vi "queue client testing.vi"() -> ()   [LabVIEW 2015]
uses:
  connection/connection maintainer.lvclass
  message/communicator message.lvclass
  Queue connection/queue pair.ctl
  message/communicator message.lvclass/communicator message.ctl
  communicator/communicator.lvclass/communicator.ctl
  Queue Client/opening handshake data.ctl
  Queue Client/Queue client.lvclass
  Queue connection/Queue connection.lvclass
  communicator/communicator.lvclass
panel:
  out "data 4":variant
  out "ID 4":string
  out "data 3":variant
  out "ID 3":string
  out "conn":refnum<class "connection maintainer.lvclass">
  out "error out 2":errorcluster
  out "listen error":errorcluster
  in  "read queue":bool
  in  "close connn":bool
  in  "listen":bool
  out "error out 4":errorcluster
  out "error out":errorcluster
  in  "send queue":bool
  in  "data 2":string
  in  "ID 2":string
  in  "data":string
  in  "ID":string
  in  "stop":bool
  in  "send handler":bool
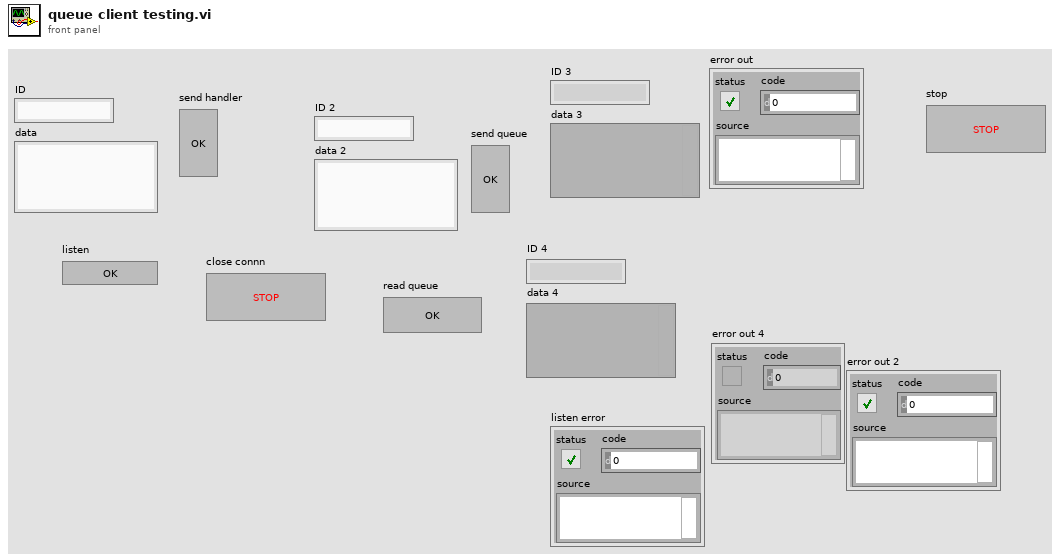
[diagram p1: front panel]
types:
  T1 = typedef "Queue connection.lvclass/queue pair.ctl" = cluster{"to pair":refnum<queue>, "from pair":refnum<queue>}
  T2 = typedef "Queue client.lvclass/opening handshake data.ctl" = cluster{"queue":refnum<queue>, "process ID":string}
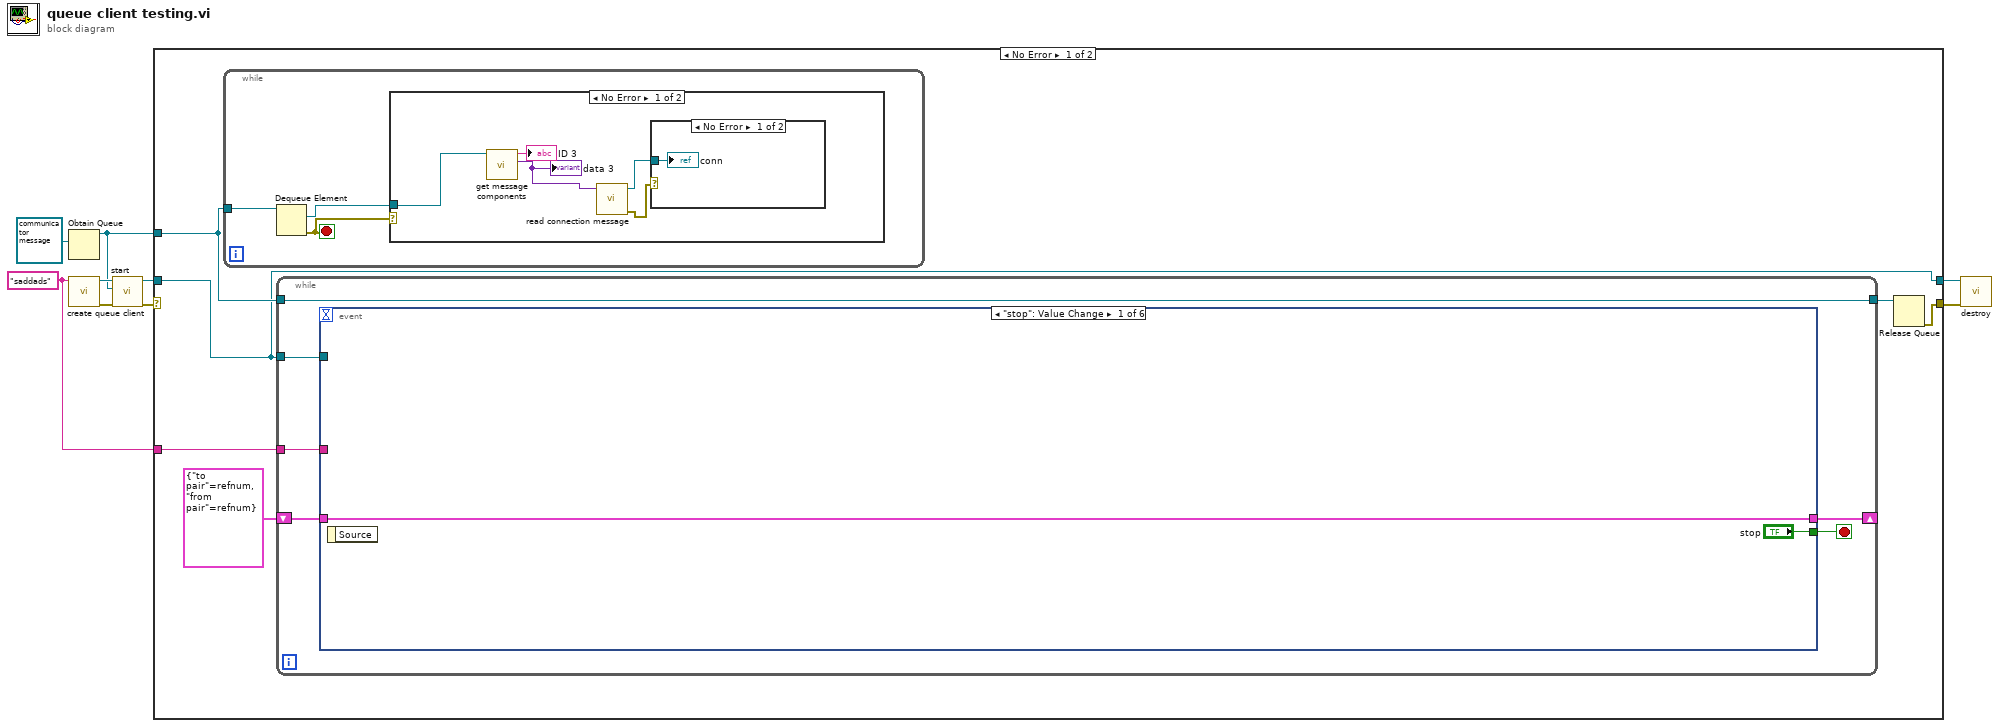
[diagram p0: block diagram]
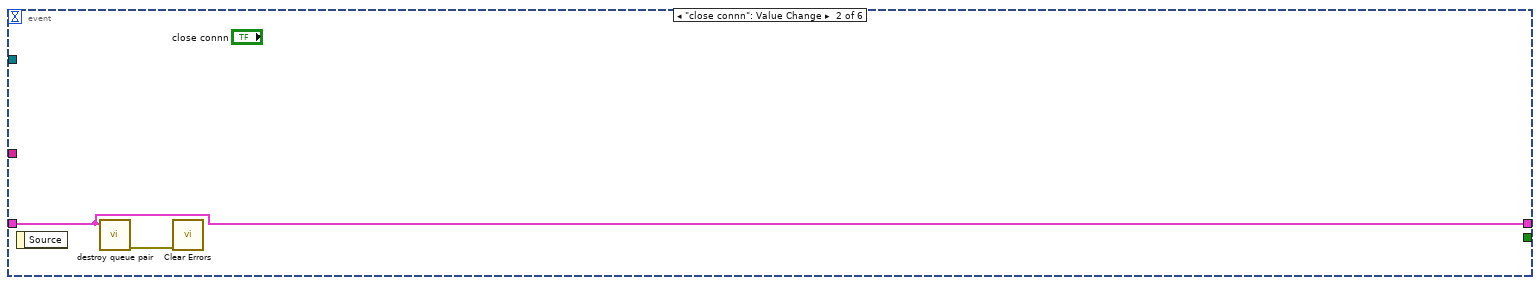
[diagram p2: hidden frame]
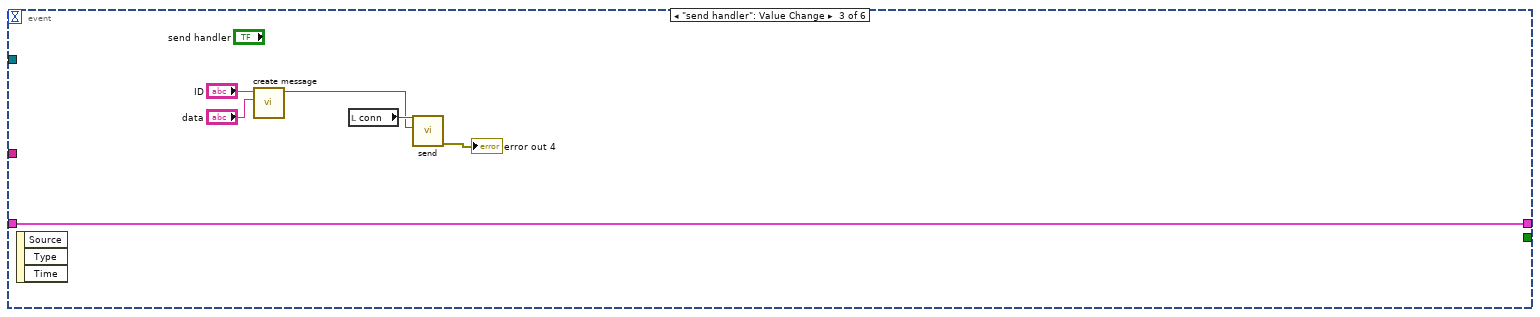
[diagram p3: hidden frame]
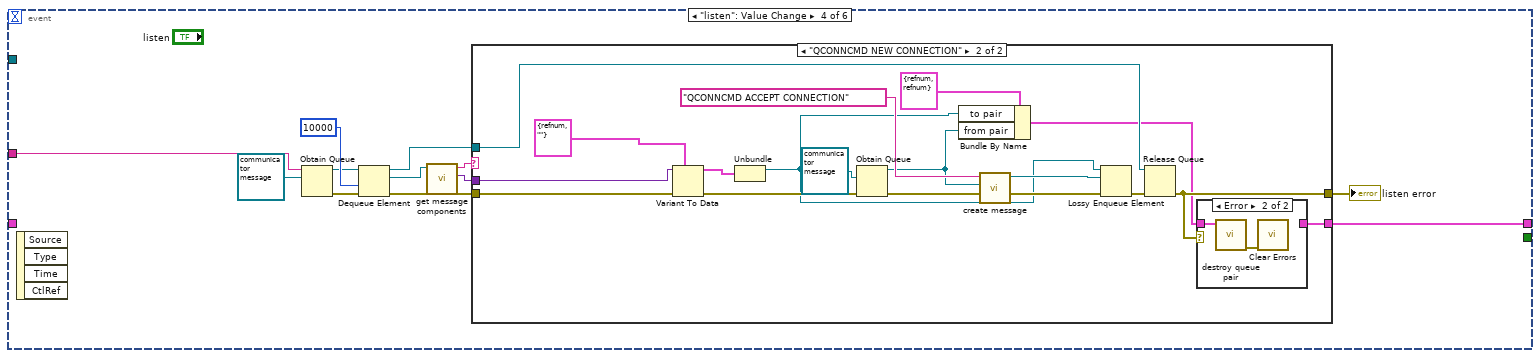
[diagram p4: hidden frame]
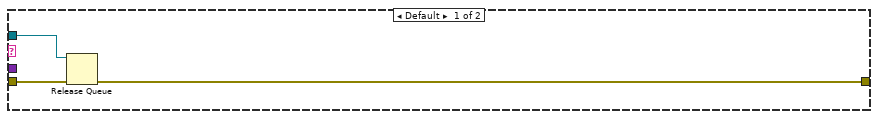
[diagram p5: hidden frame]
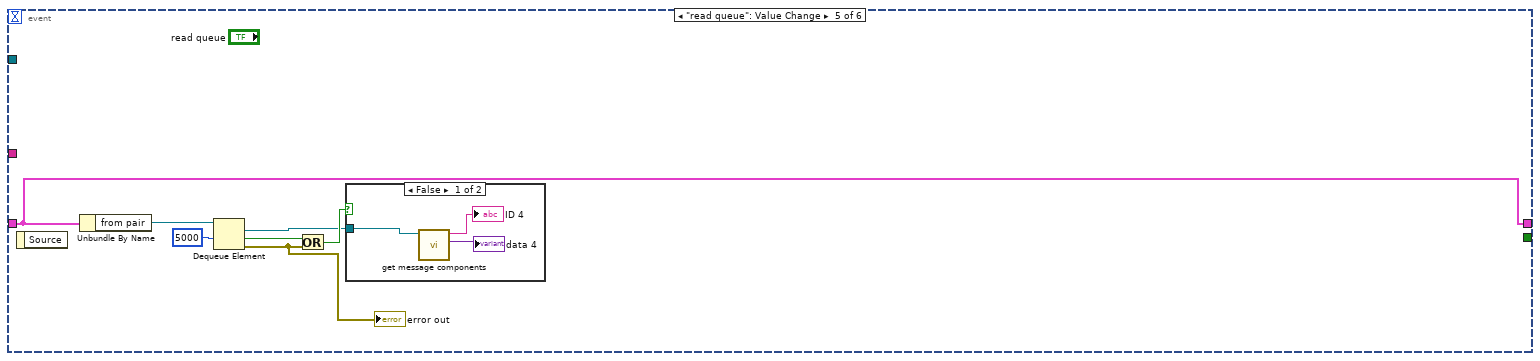
[diagram p7: hidden frame]
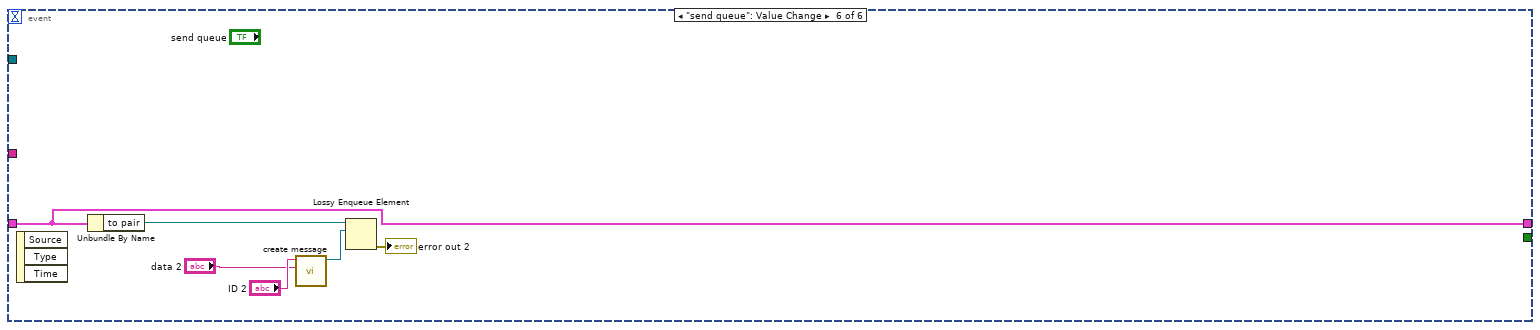
[diagram p9: hidden frame]
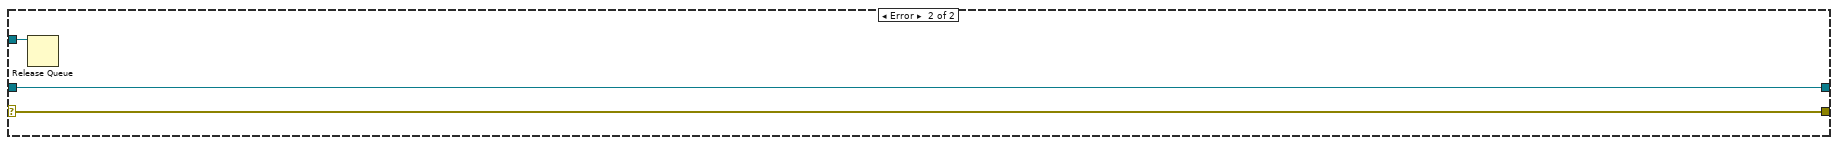
[diagram p12: hidden frame]
diagram:
  w1 = "saddads" ("connection string")
  n1 = Obtain Queue(element data type=refnum<class "communicator message.lvclass"> refnum ("communicator message.lvclass")) -> (queue out=w4:refnum<queue>)  [unwired: 4 in, 2 out]
  n2 = call "create queue client.vi"("conn string"=w1) -> ("error out"=w5:errorcluster, "TCP client out"=w6:refnum<class "Queue client.lvclass">)  [unwired: 9 in]
  n3 = call-dynamic "start.vi"("error in"=w5, "queue to parent"=w4, "communicator in"=w6) -> ("error out"=w2:errorcluster, "communicator out"=w3:refnum<class "Queue client.lvclass">)  [unwired: 7 in]
  n4 = case shown="No Error" w2 {
    selector: w2 -> [_ w94]
    tunnel: [w12 w92] -> w8
    tunnel: w4 -> [w15 w93]
    tunnel: [w13 w94] -> w7
    tunnel: w3 -> [w12 w92]
    tunnel: w1 -> [w10 _]
    frame No Error {
      n5 = while {
        tunnel: w15 -> [w85]
        stop <- w83 stop-if-true
        n6 = Dequeue Element(queue=w85) -> (element=w84:refnum<class "communicator message.lvclass">, error out=w83:errorcluster)  [unwired: 2 in, 2 out]
        n7 = case shown="No Error" w83 {
          tunnel: w84 -> [w88 _]
          frame No Error {
            n8 = call "get message components.vi"("message"=w88) -> ("data"=w87:variant, "ID"=→"ID 3":string)  [unwired: 9 in]
            "data 3" <- w87
            n9 = call "read connection message.vi"("data"=w87) -> ("error out"=w89:errorcluster, "conn"=w90:refnum<class "connection maintainer.lvclass">)  [unwired: 9 in]
            n10 = case shown="No Error" w89 {
              tunnel: w90 -> [w91 _]
              frame No Error {
                "conn" <- w91
              }
              frame Error {
              }
            }
          }
          frame Error {
          }
        }
      }
      n11 = while {
        tunnel: w12 -> [w19]
        tunnel: [w20] -> w14
        tunnel: w15 -> [w20]
        shift-right: [w18] -> _
        shift-left: T1 {"to pair"=refnum, "from pair"=refnum} ("output cluster 2") -> [w17]
        tunnel: w10 -> [w16]
        stop <- w21 stop-if-true
        n12 = event shown="[0] \"stop\": Value Change" {
          selector: _ -> [_ _ _ _ _ _]
          dyn-events: _ -> [_ _ _ _ _ _]
          timeout: _ -> [_ _ _ _ _ _]
          tunnel: ["stop" _ _ _ _ _] -> w21
          tunnel: w19 -> [_ _ _ _ _ _]
          tunnel: [w22 w24 w31 w36 w73 w82] -> w18
          tunnel: w17 -> [w22 w24 w31 _ w73 w82]
          tunnel: w16 -> [_ _ _ w35 _ _]
          event "stop": Value Change {
            n13 = event-data() -> ()  [unwired: 1 in, 1 out]
          }
          event "close connn": Value Change {
            n14 = event-data() -> ()  [unwired: 1 in, 1 out]
            n15 = call "destroy queue pair.vi"("queue connection"=w24) -> ("error out"=w25:errorcluster)  [unwired: 10 in]
            n16 = call <vilib>:"Clear Errors.vi"("error in (no error)"=w25) -> ()  [unwired: 5 in, 2 out]
          }
          event "send handler": Value Change {
            n17 = event-data() -> ()  [unwired: 1 in, 3 out]
            n18 = call "create message.vi"("data"="data", "ID"="ID") -> ("message"=w26:refnum<class "communicator message.lvclass">)  [unwired: 9 in]
            n19 = local read "conn"() -> (w30:refnum<class "connection maintainer.lvclass">)
            n20 = call "send.vi"("element"=w26, "communicator in"=w30) -> ("error out"=→"error out 4":errorcluster)  [unwired: 9 in]
          }
          event "listen": Value Change {
            n21 = event-data() -> ()  [unwired: 1 in, 4 out]
            n22 = Obtain Queue(name (unnamed)=w35, element data type=refnum<class "communicator message.lvclass"> refnum ("communicator message.lvclass")) -> (queue out=w39:refnum<queue>, error out=w42:errorcluster)  [unwired: 3 in, 1 out]
            n23 = Dequeue Element(queue=w39, timeout in ms (-1)=10000 ("timeout ms (60000)"), error in (no error)=w42) -> (queue out=w38:refnum<queue>, element=w32:refnum<class "communicator message.lvclass">, error out=w41:errorcluster)  [unwired: 1 out]
            n24 = call "get message components.vi"("message"=w32) -> ("data"=w33:variant, "ID"=w34:string)  [unwired: 9 in]
            n25 = case shown="\"QCONNCMD NEW CONNECTION\"" w34 {
              tunnel: w41 -> [w46 w63]
              tunnel: w38 -> [w45 w58]
              tunnel: [w44 w56] -> w37
              tunnel: w33 -> [_ w62]
              tunnel: [_ w54] -> w36
              frame Default {
                n26 = Release Queue(queue=w45, error in (no error)=w46) -> (error out=w44:errorcluster)  [unwired: 1 in, 2 out]
              }
              frame "QCONNCMD NEW CONNECTION" {
                n27 = Variant To Data(error in=w63, type=T2 {"queue"=refnum, "process ID"=""} ("handshake data"), Variant=w62) -> (data=w53:T2, error out=w60:errorcluster)
                n28 = Unbundle(w53) -> ("queue"=w47:refnum<queue>)  [unwired: 1 out]
                n29 = Obtain Queue(element data type=refnum<class "communicator message.lvclass"> refnum ("communicator message.lvclass"), error in (no error)=w60) -> (queue out=w50:refnum<queue>, error out=w52:errorcluster)  [unwired: 3 in, 1 out]
                n30 = Bundle By Name(cluster=T1 {"to pair"=refnum, "from pair"=refnum} ("queues"), "to pair"=w47, "from pair"=w50) -> (w55:T1)
                n31 = call "create message.vi"("data"=w50, "ID"="QCONNCMD ACCEPT CONNECTION") -> ("message"=w49:refnum<class "communicator message.lvclass">)  [unwired: 9 in]
                n32 = Lossy Enqueue Element(queue=w47, element=w49, error in (no error)=w52) -> (error out=w57:errorcluster)  [unwired: 3 out]
                n33 = Release Queue(queue=w58, error in (no error)=w57) -> (error out=w56:errorcluster)  [unwired: 1 in, 2 out]
                n34 = case shown="Error" w56 {
                  tunnel: w55 -> [w64 w66]
                  tunnel: [w64 _] -> w54
                  frame No Error {
                  }
                  frame Error {
                    n35 = call "destroy queue pair.vi"("queue connection"=w66) -> ("error out"=w65:errorcluster)  [unwired: 10 in]
                    n36 = call <vilib>:"Clear Errors.vi"("error in (no error)"=w65) -> ()  [unwired: 5 in, 2 out]
                  }
                }
              }
            }
            "listen error" <- w37
          }
          event "read queue": Value Change {
            n37 = event-data() -> ()  [unwired: 1 in, 1 out]
            n38 = Unbundle By Name(w73) -> ("from pair"=w72:refnum<queue>)
            n39 = Dequeue Element(queue=w72, timeout in ms (-1)=5000) -> (element=w68:refnum<class "communicator message.lvclass">, timed out?=w70:bool, error out=w67:errorcluster)  [unwired: 1 in, 1 out]
            "error out" <- w67
            n40 = Or(x=w70, y=w67) -> (x .or. y?=w69:bool)
            n41 = case shown="False" w69 {
              tunnel: w68 -> [w76 _]
              frame False {
                n42 = call "get message components.vi"("message"=w76) -> ("data"=→"data 4":variant, "ID"=→"ID 4":string)  [unwired: 9 in]
              }
              frame True {
              }
            }
          }
          event "send queue": Value Change {
            n43 = event-data() -> ()  [unwired: 1 in, 3 out]
            n44 = Unbundle By Name(w82) -> ("to pair"=w81:refnum<queue>)
            n45 = call "create message.vi"("data"="data 2", "ID"="ID 2") -> ("message"=w78:refnum<class "communicator message.lvclass">)  [unwired: 9 in]
            n46 = Lossy Enqueue Element(queue=w81, element=w78) -> (error out=→"error out 2":errorcluster)  [unwired: 1 in, 3 out]
          }
        }
      }
      n47 = Release Queue(queue=w14) -> (error out=w13:errorcluster)  [unwired: 2 in, 2 out]
    }
    frame Error {
      n48 = Release Queue(queue=w93) -> ()  [unwired: 2 in, 3 out]
    }
  }
  n49 = call-dynamic "destroy.vi"("error in"=w7, "communicator in"=w8) -> ()  [unwired: 9 in, 1 out]
